vi "ARC_Queue Remove Element.vi"(7 "Time out(-1)_queue out":i32=-1 caption="Time Out(-1)_Queue Out", 8 "error in (no error)":errorcluster caption="Error In (no error)", 11 "Queue Name(unamed)":string) -> (0 "error out":errorcluster caption="Error Out", 1 "timed out":bool caption="Time Out?", 2 "Data":variant, 3 "Event":string)   [LabVIEW 2016]
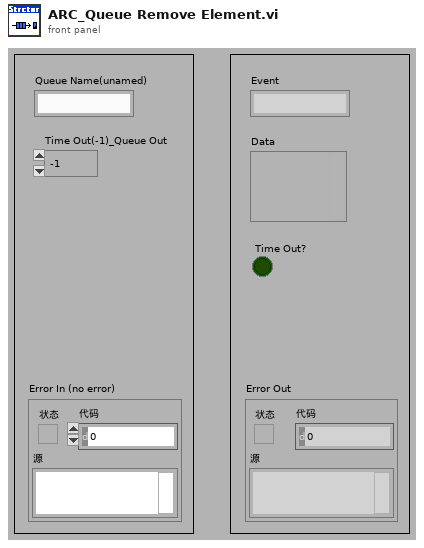
[diagram p1: front panel]
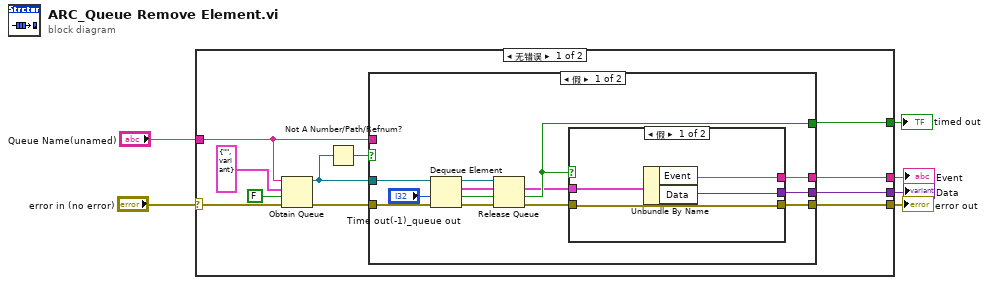
[diagram p0: block diagram]
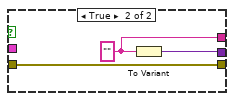
[diagram p2: hidden frame]
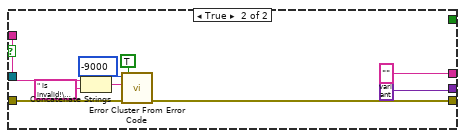
[diagram p3: hidden frame]
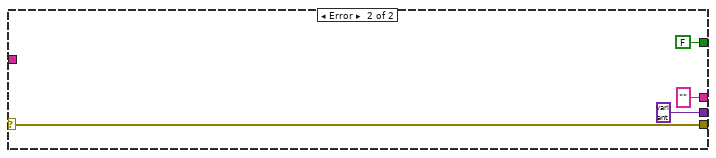
[diagram p4: hidden frame]
diagram:
  n1 = case shown="无错误" "error in (no error)" {
    selector: "error in (no error)" -> [w12 w48]
    tunnel: [w17 w48] -> w5
    tunnel: "Queue Name(unamed)" -> [w11 _]
    tunnel: [w9 variant ("Variant")] -> w3
    tunnel: [w8 "" ("Command 2")] -> w2
    tunnel: [w7 FALSE ("timed out?")] -> w1
    frame No Error {
      n2 = Obtain Queue(name (unnamed)=w11, element data type=cluster{"Event":string, "Data":variant} {"Event"="", "Data"=variant} ("输出簇"), create if not found? (T)=FALSE ("如未找到是否创建？(T)"), error in (no error)=w12) -> (queue out=w14:refnum<queue>, error out=w13:errorcluster)  [unwired: 1 in, 1 out]
      n3 = Not A Number/Path/Refnum?(number/path/refnum=w14) -> (NaN/Path/Refnum?=w15:bool)
      n4 = case shown="假" w15 {
        tunnel: [w28 variant ("Variant")] -> w9
        tunnel: [w27 "" ("Command 2")] -> w8
        tunnel: w13 -> [w24 w38]
        tunnel: [w26 w37] -> w17
        tunnel: [w22 _] -> w7
        tunnel: w11 -> [_ w36]
        tunnel: w14 -> [w25 _]
        frame False {
          n5 = Dequeue Element(queue=w25, timeout in ms (-1)="Time out(-1)_queue out", error in (no error)=w24) -> (queue out=w19:refnum<queue>, element=w21:cluster{"Event":string, "Data":variant}, timed out?=w22:bool, error out=w20:errorcluster)
          n6 = Release Queue(queue=w19, error in (no error)=w20) -> (error out=w18:errorcluster)  [unwired: 1 in, 2 out]
          n7 = case shown="假" w22 {
            tunnel: w21 -> [w29 _]
            tunnel: [w32 w35] -> w28
            tunnel: [w31 w34] -> w27
            tunnel: w18 -> [w30 w33]
            tunnel: [w30 w33] -> w26
            frame False {
              n8 = Unbundle By Name(w29) -> ("Event"=w31:string, "Data"=w32:variant)
            }
            frame True {
              w34 = "" ("Command 2")
              n9 = To Variant(anything=w34) -> (Variant=w35:variant)
            }
          }
        }
        frame True {
          n10 = Concatenate Strings(w36, " is invalid!\nEnsure the queue has been created!" ("字符串")) -> (w41:string)
          n11 = call <vilib>:"Error Cluster From Error Code.vi"("show call chain? (False)"=TRUE, "error in (no error)"=w38, "error message (\"\")"=w41, "error code (0)"=-9000) -> ("error out"=w37:errorcluster)  [unwired: 5 in]
        }
      }
    }
    frame Error {
    }
  }
  "error out" <- w5
  "Event" <- w2
  "Data" <- w3
  "timed out" <- w1
